vi "Is Null.vi"(1 "Value in":variant) -> (0 "Is Value Null?":bool)   [LabVIEW 2019, in "JSON.lvlib"]
doc: "Returns <b>True</b> if the <b>Value in</b> is the U8 Enum \"<b>null</b>\" placeholder.\n\nCreated by: Ryan Pacini"
uses:
  JSON.lvlib
  <vilib>/Utility/Data Type/NI_Data Type.lvlib
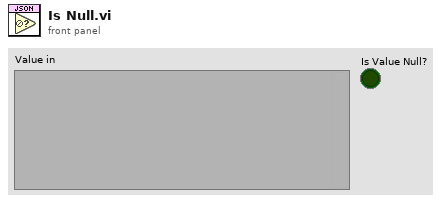
[diagram p1: front panel]
types:
  T1 = typedef "NI_Data Type.lvlib/Data Type.ctl" = enum8{"Invalid Type", "Void", "I8", "I16", "I32", "I64", "U8", "U16", "U32", "U64", "Single Float", "Double Float", "Extended Float", "Single Complex", "Double Complex", "Extended Complex", "Enum U8", "Enum U16", "Enum U32", "Enum U64", "Single Float With Unit", "Double Float With Unit", "Extended Float With Unit", "Single Complex with Unit", "Double Complex with Unit", "Extended Complex with Unit", "Boolean", "String", "Path", "Picture", "Tag", "Array", "Cluster", "Variant", "LV Variant", "Waveform", "Timestamp", "Digital Waveform", "Digital Data", "ExpressData", "Refnum", "External Data", "VI", "Poly VI", "LabVIEW Class Instance", "Fixed Point", "Set Collection", "Map Collection"}
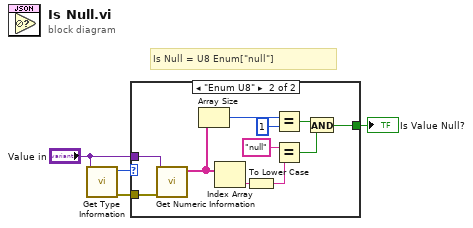
[diagram p0: block diagram]
diagram:
  # "Is Null = U8 Enum[\"null\"]"
  n1 = call <vilib>:"Get Type Information.vi"("variant"="Value in") -> ("error out"=w3:errorcluster, "type"=w4:T1)  [unwired: 6 in, 3 out]
  n2 = case shown="\"Enum U8\"" w4 {
    tunnel: w3 -> [_ w15]
    tunnel: "Value in" -> [_ w14]
    tunnel: [_ w5] -> w1
    frame "Invalid Type", Default {
    }
    frame "Enum U8" {
      n3 = call <vilib>:"Get Numeric Information.vi"("error in (no error)"=w15, "variant"=w14) -> ("enum names"=w11:string[])  [unwired: 6 in, 3 out]
      n4 = Array Size(array=w11) -> (size(s)=w13:i32)
      n5 = Index Array(array=w11) -> (element=w10:string)  [unwired: 1 in]
      n6 = To Lower Case(string=w10) -> (all lower case string=w8:string)
      n7 = Equal?(x=w13, y=1) -> (x = y?=w6:bool)
      n8 = Equal?(x="null" ("y"), y=w8) -> (x = y?=w7:bool)
      n9 = And(x=w6, y=w7) -> (x .and. y?=w5:bool)
    }
  }
  "Is Value Null?" <- w1
